vi "Stepper Drive Publish Messages.vi"(8 "error in (no error)":errorcluster, 9 "Parameter":string, 10 "Message":string, 11 "Axis Config Constant":T1) -> ()   [LabVIEW 2016, in "SMD-7615.lvlib"]
uses:
  SMD-7615.lvlib
  CTL/Stepper Drive Config.ctl
  CTL/SV General.ctl
  CTL/SV Inputs.ctl
  CTL/SV Outputs.ctl
  LUL-All/LUL-Syslog/LUL-SysLog.lvlib
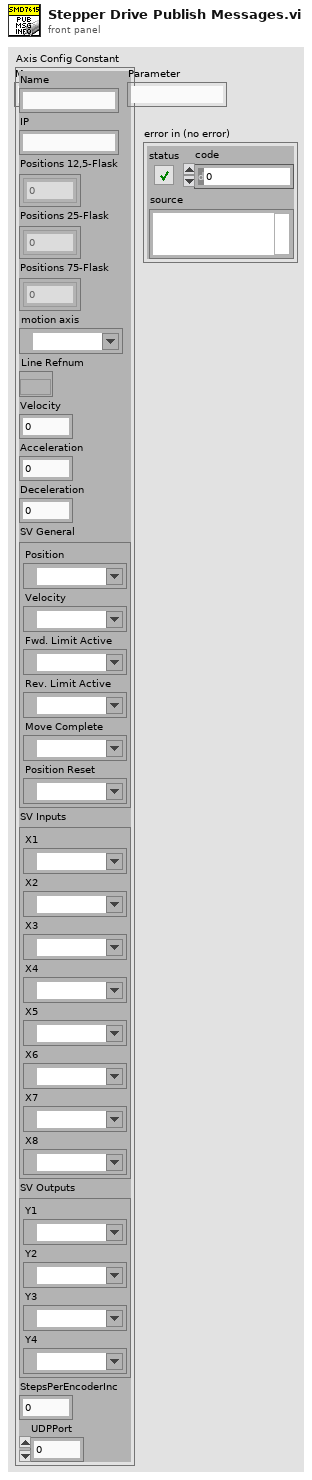
[diagram p1: front panel]
types:
  T1 = typedef "SMD-7615.lvlib/Stepper Drive Config.ctl" = cluster{"Name":string, "IP":string, "Positions 12,5-Flask":dbl[], "Positions 25-Flask":dbl[], "Positions 75-Flask":dbl[], "motion axis ":refnum<k21>, "Line Refnum":refnum<k20>, "Velocity":dbl, "Acceleration":dbl, "Deceleration":dbl, "SV General":T2, "SV Inputs":T3, "SV Outputs":T4, "StepsPerEncoderInc":i32, "UDPPort":u16}
  T2 = typedef "SMD-7615.lvlib/SV General.ctl" = cluster{"Position":refnum<k21>, "Velocity":refnum<k21>, "Fwd. Limit Active":refnum<k21>, "Rev. Limit Active":refnum<k21>, "Move Complete":refnum<k21>, "Position Reset":refnum<k21>}
  T3 = typedef "SMD-7615.lvlib/SV Inputs.ctl" = cluster{"X1":refnum<k21>, "X2":refnum<k21>, "X3":refnum<k21>, "X4":refnum<k21>, "X5":refnum<k21>, "X6":refnum<k21>, "X7":refnum<k21>, "X8":refnum<k21>}
  T4 = typedef "SMD-7615.lvlib/SV Outputs.ctl" = cluster{"Y1":refnum<k21>, "Y2":refnum<k21>, "Y3":refnum<k21>, "Y4":refnum<k21>}
  T5 = typedef "LUL-SysLog.lvlib/SysLog Severity.ctl" = enum16{"Emergency", "Alert", "Critical", "Error", "Wanring", "Notice", "Informational", "Debug"}
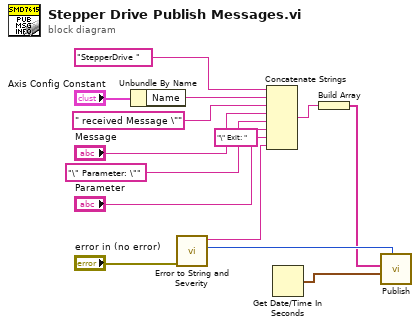
[diagram p0: block diagram]
diagram:
  n1 = Unbundle By Name("Axis Config Constant") -> ("Name"=w13:string)
  n2 = call "Error to String and Severity.vi"("error in (no error)"="error in (no error)") -> ("Severity"=w7:T5, "Error Text"=w1:string)  [unwired: 9 in]
  n3 = Concatenate Strings("StepperDrive " ("string"), w13, " received Message \"" ("string"), "Message", "\" Parameter: \"" ("string"), "Parameter", "\" Exit: " ("string"), w1) -> (w6:string)
  n4 = Get Date/Time In Seconds() -> (seconds since 1Jan1904=w12:timestamp)
  n5 = Build Array(w6) -> (w5:string[])
  n6 = call "Publish.vi"("Severity"=w7, "current time"=w12, "Message"=w5) -> ()  [unwired: 8 in, 1 out]
